vi "timeoutCheckStatus.vi"(8 "error in (no error)":errorcluster, 11 "GiaoTiepUART in":refnum<class "GiaoTiepUART.lvclass">) -> (0 "error out":errorcluster, 3 "GiaoTiepUART out":refnum<class "GiaoTiepUART.lvclass">)   [LabVIEW 2017, in "GiaoTiepUART.lvclass"]
uses:
  GiaoTiepUART.lvclass
  GiaoTiepUART.lvclass/GiaoTiepUART.ctl
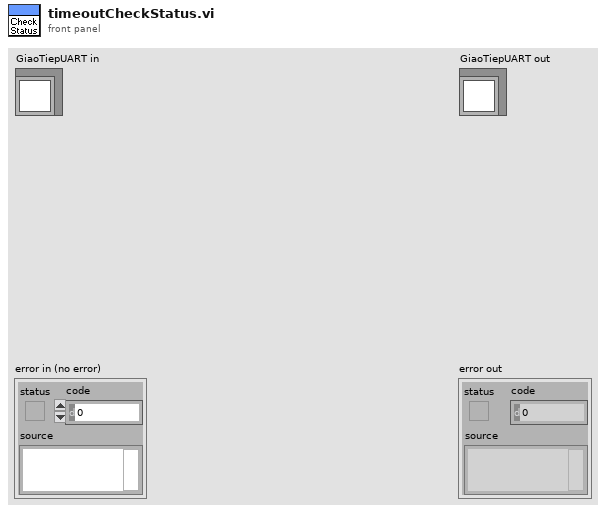
[diagram p1: front panel]
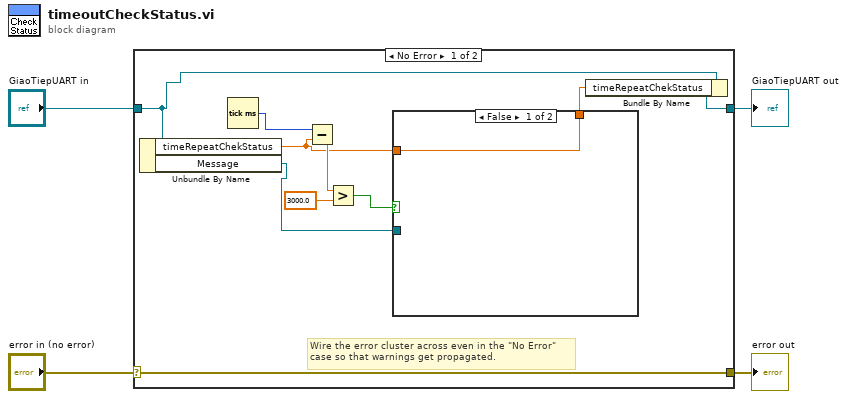
[diagram p0: block diagram]
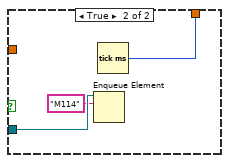
[diagram p2: hidden frame]
diagram:
  n1 = case shown="No Error" "error in (no error)" {
    selector: "error in (no error)" -> [w14 w20]
    tunnel: [w14 w20] -> w3
    tunnel: [w7 w19] -> w1
    tunnel: "GiaoTiepUART in" -> [w8 w19]
    frame No Error {
      # "Wire the error cluster across even in the \"No Error\"\ncase so that warnings get propagated."
      n2 = Unbundle By Name(w8) -> ("timeRepeatChekStatus"=w5:dbl, "Message"=w9:refnum<queue>)
      n3 = Tick Count (ms)() -> (millisecond timer value=w13:u32)
      n4 = Subtract(x=w13, y=w5) -> (x-y=w12:dbl)
      n5 = Greater?(x=w12, y=3000.0) -> (0:w10:bool)
      n6 = case shown="False" w10 {
        tunnel: w9 -> [_ w18]
        tunnel: [w15 w16] -> w6
        tunnel: w5 -> [w15 _]
        frame False {
        }
        frame True {
          n7 = Enqueue Element(queue=w18, element="M114") -> ()  [unwired: 2 in, 3 out]
          n8 = Tick Count (ms)() -> (millisecond timer value=w16:u32)
        }
      }
      n9 = Bundle By Name(cluster=w8, "timeRepeatChekStatus"=w6) -> (w7:refnum<class "GiaoTiepUART.lvclass">)
    }
    frame Error {
    }
  }
  "error out" <- w3
  "GiaoTiepUART out" <- w1
